vi "hoofdprogramma.vi"   [LabVIEW 2019]
uses:
  <vilib>/myRIO/Common/Instrument Driver Framework/Utilities/typedefs/Analog Scaling Constants.ctl
  <vilib>/myRIO/Common/Instrument Driver Framework/Utilities/typedefs/Analog Scaling Constants List.ctl
  <vilib>/myRIO/Common/Instrument Driver Framework/myRIO v1.0/AO/typedefs/AO Channels Enum.ctl
  <vilib>/myRIO/Common/Instrument Driver Framework/myRIO v1.0/AO/typedefs/AO Channels List.ctl
  <vilib>/myRIO/Common/Instrument Driver Framework/Utilities/typedefs/Generic FPGA Reference.ctl
  <vilib>/myRIO/Common/Instrument Driver Framework/Utilities/typedefs/myRIO v1.0 Reference.ctl
  <vilib>/myRIO/Common/Instrument Driver Framework/Utilities/typedefs/Hardware Version Enum.ctl
  <vilib>/myRIO/Common/Instrument Driver Framework/Utilities/typedefs/myRIO Generic Hardware Reference.ctl
  <vilib>/myRIO/Instrument Drivers/Onboard IO/AO/typedefs/AO Reference.ctl
  <vilib>/myRIO/Instrument Drivers/Onboard IO/AO/AO.lvlib
  <vilib>/myRIO/Instrument Drivers/Onboard IO/AO/vis/Write.vi
  <vilib>/userDefined/High Color/nirio_resource_hc.ctl
  <vilib>/myRIO/Common/Instrument Driver Framework/myRIO v1.0/AO/vis/myRIO v1.1 Open AO.vi
  <vilib>/myRIO/Instrument Drivers/Onboard IO/AO/vis/myRIO AO Open.xnode
  <vilib>/myRIO/Common/Instrument Driver Framework/Utilities/vis/Is FPGA Ref Available.vi
  <vilib>/myRIO/Express VI/Onboard IO/AO/AO Express VI.xnode
  <vilib>/myRIO/Common/Instrument Driver Framework/myRIO v1.0/DIO/typedefs/DIO Channels Enum.ctl
  <vilib>/myRIO/Common/Instrument Driver Framework/myRIO v1.0/DIO/typedefs/DIO Channels List.ctl
  <vilib>/myRIO/Instrument Drivers/Onboard IO/DIO/typedefs/DIO Reference.ctl
  <vilib>/myRIO/Instrument Drivers/Onboard IO/DIO/DIO.lvlib
  <vilib>/myRIO/Instrument Drivers/Onboard IO/DIO/vis/myRIO DIO Open.xnode
  <vilib>/myRIO/Common/Instrument Driver Framework/myRIO v1.0/DIO/vis/myRIO v1.1 Open DIO.vi
  <vilib>/myRIO/Instrument Drivers/Onboard IO/DIO/vis/Write.vi
  <vilib>/myRIO/Express VI/Onboard IO/DO/DO Express VI.xnode
  <vilib>/myRIO/Express VI/Onboard IO/DI/DI Express VI.xnode
  <vilib>/myRIO/Instrument Drivers/Onboard IO/DIO/vis/Read.vi
  interface.vi
types:
  T1 = typedef "DIO.lvlib/DIO Reference.ctl" = cluster{"myRIO Reference":T2, "DIO Channels List":T6}
  T2 = typedef "myRIO Generic Hardware Reference.ctl" = cluster{"myRIO Model":T3, "myRIO Hardware Reference":T4}
  T3 = typedef "Hardware Version Enum.ctl" = enum16{"Unknown", "myRIO-1900", "myRIO-1950", "roboRIO", "NI ELVIS RIO CM", "ELVIS III"}
  T4 = typedef "myRIO v1.0 Reference.ctl" = cluster{"Generic FPGA Reference":T5, "Allow multiple opens":bool}
  T5 = typedef "Generic FPGA Reference.ctl" = refnum<k20>
  T6 = typedef "DIO Channels List.ctl" = T7[]
  T7 = typedef "DIO Channels Enum.ctl" = enum16{"Not Connected", "C/DIO0", "C/DIO1", "C/DIO2", "C/DIO3", "C/DIO4", "C/DIO5", "C/DIO6", "C/DIO7", "A/DIO0", "A/DIO1", "A/DIO2", "A/DIO3", "A/DIO4", "A/DIO5", "A/DIO6", "A/DIO7", "A/DIO8", "A/DIO9", "A/DIO10", "A/DIO11", "A/DIO12", "A/DIO13", "A/DIO14", "A/DIO15", "A/DIO16", "A/DIO17", "A/DIO18", "A/DIO19", "B/DIO0", "B/DIO1", "B/DIO2", "B/DIO3", "B/DIO4", "B/DIO5", "B/DIO6", "B/DIO7", "B/DIO8", "B/DIO9", "B/DIO10", "B/DIO11", "B/DIO12", "B/DIO13", "B/DIO14", "B/DIO15", "B/DIO16", "B/DIO17", "B/DIO18", "B/DIO19", "LED0", "LED1", "LED2", "LED3", "Button0", "DIO/DIO0", "DIO/DIO1", "DIO/DIO2", "DIO/DIO3", "DIO/DIO4", "DIO/DIO5", "DIO/DIO6", "DIO/DIO7", "DIO/DIO8", "DIO/DIO9", "SPI/CS0", "SPI/CS1", "SPI/CS2", "SPI/CS3", "LED RADIO (Green)", "LED RADIO (Red)", "LED COMM (Green)", "LED COMM (Red)", "LED MODE (Green)", "LED MODE (Red)"}
  T8 = typedef "nirio_resource_hc.ctl" = tag
  T9 = typedef "AO.lvlib/AO Reference.ctl" = cluster{"myRIO Reference":T2, "AO Channel List":T10, "AO Scaling Constant List":T12}
  T10 = typedef "AO Channels List.ctl" = T11[]
  T11 = typedef "AO Channels Enum.ctl" = enum16{"Not Connected", "AudioOut/Left", "AudioOut/Right", "C/AO0", "C/AO1", "A/AO0", "A/AO1", "B/AO0", "B/AO1"}
  T12 = typedef "Analog Scaling Constants List.ctl" = T13[]
  T13 = typedef "Analog Scaling Constants.ctl" = cluster{"LSB Weight (Volts)":dbl, "Offset (Volts)":dbl, "Signed?":bool}
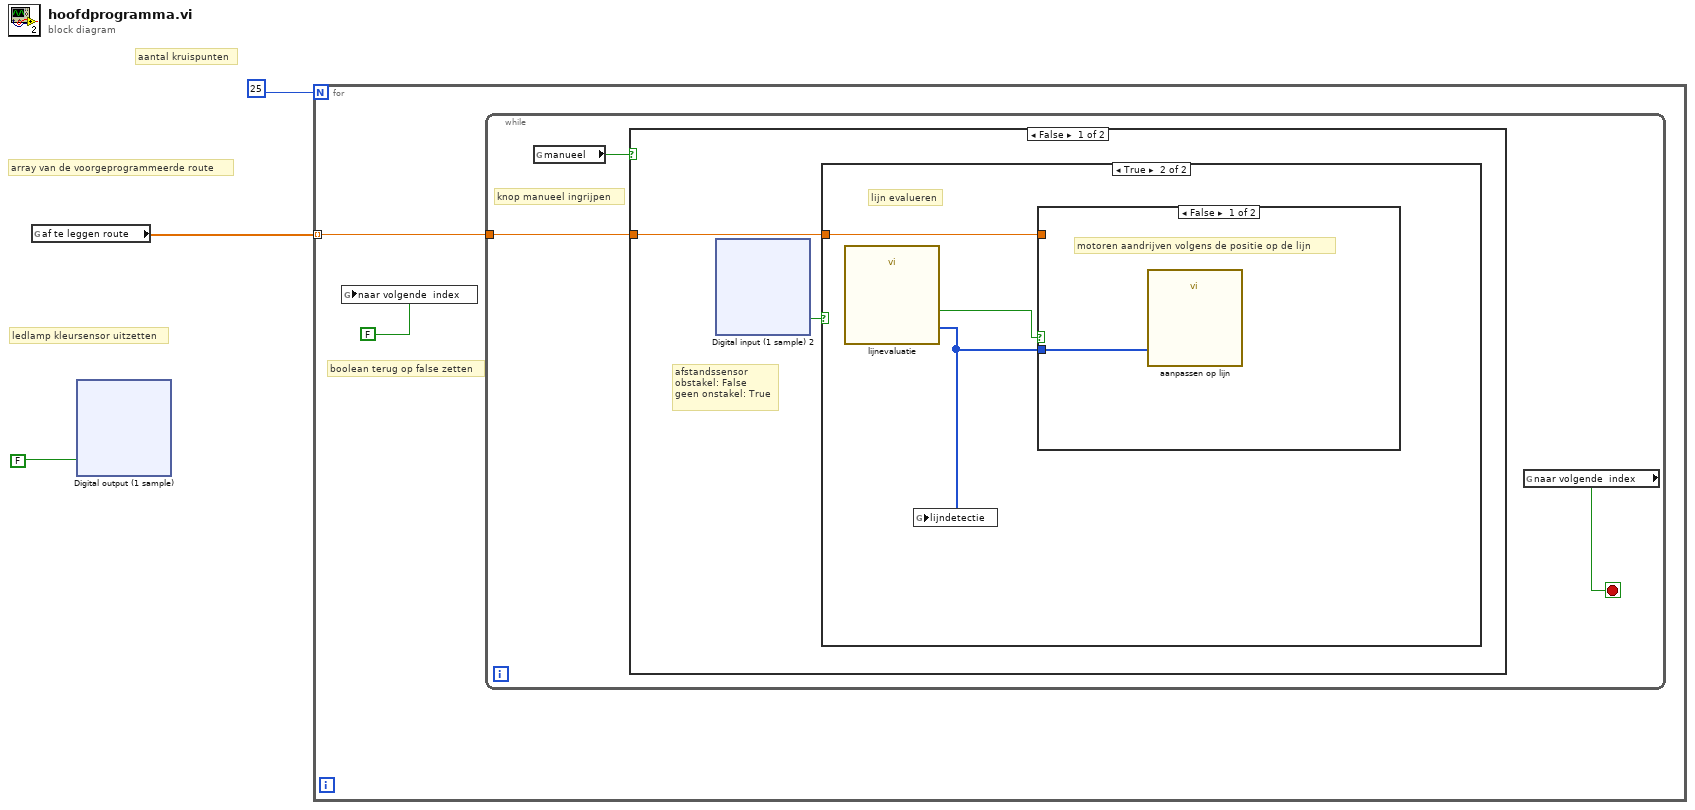
[diagram p0: block diagram]
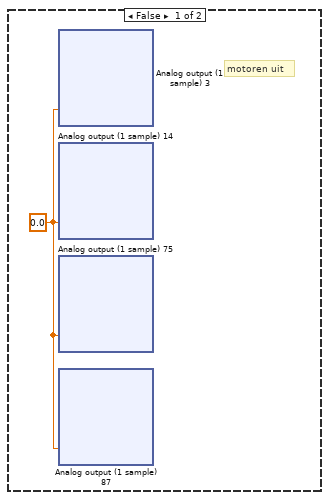
[diagram p2: hidden frame]
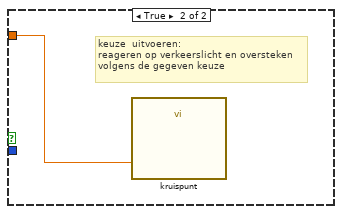
[diagram p3: hidden frame]
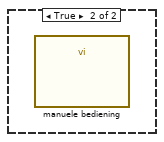
[diagram p4: hidden frame]
diagram:
  # "array van de voorgeprogrammeerde route"
  # "aantal kruispunten"
  # "ledlamp kleursensor uitzetten"
  n1 = global read "interface.vi" "af te leggen route"() -> (w1:dbl[])
  n2 = xnode "Digital output (1 sample)"("A/DIO2 (Pin 15)"=FALSE) -> ()  [unwired: 1 in, 1 out]
  n3 = for {
    N: 25 -> [_]
    tunnel: w1 -> [w5] mode=indexing
    # "boolean terug op false zetten"
    n4 = global write "interface.vi" "naar volgende  index"(FALSE) -> ()
    n5 = while {
      tunnel: w5 -> [w8]
      stop <- w6 stop-if-true
      # "knop manueel ingrijpen"
      n6 = global read "interface.vi" "manueel"() -> (w7:bool)
      n7 = case shown="False" w7 {
        tunnel: w8 -> [w9 _]
        frame False {
          # "afstandssensor\nobstakel: False\ngeen onstakel: True"
          n8 = xnode "Digital input (1 sample) 2"() -> ("A/DIO1 (Pin 13)"=w10:bool)  [unwired: 1 in, 1 out]
          n9 = case shown="True" w10 {
            tunnel: w9 -> [_ w197]
            frame False {
              w46 = 0.0
              # "motoren uit"
              n10 = xnode "Analog output (1 sample) 3"("A/AO0 (Pin 2)"=w46) -> ()  [unwired: 1 in, 1 out]
              n11 = xnode "Analog output (1 sample) 14"("A/AO1 (Pin 4)"=w46) -> ()  [unwired: 1 in, 1 out]
              n12 = xnode "Analog output (1 sample) 75"("B/AO0 (Pin 2)"=w46) -> ()  [unwired: 1 in, 1 out]
              n13 = xnode "Analog output (1 sample) 87"("B/AO1 (Pin 4)"=w46) -> ()  [unwired: 1 in, 1 out]
            }
            frame True {
              # "lijn evalueren"
              n14 = call "lijnevaluatie.vi"() -> ("digitaal lijn 0-1"=w195:i32[], "stopstreep indicator"=w196:bool)  [unwired: 8 in, 2 out]
              n15 = global write "interface.vi" "lijndetectie"(w195) -> ()
              n16 = case shown="False" w196 {
                tunnel: w197 -> [_ w199]
                tunnel: w195 -> [w198 _]
                frame False {
                  # "motoren aandrijven volgens de positie op de lijn"
                  n17 = call "aanpassen op lijn.vi"("digitaal lijn"=w198) -> ()  [unwired: 10 in, 1 out]
                }
                frame True {
                  # "keuze  uitvoeren:\nreageren op verkeerslicht en oversteken\nvolgens de gegeven keuze"
                  n18 = call "kruispunt.vi"("keuze 1,2 of 3"=w199) -> ()  [unwired: 11 in]
                }
              }
            }
          }
        }
        frame True {
          n19 = call "manuele bediening.vi"() -> ()  [unwired: 12 in]
        }
      }
      n20 = global read "interface.vi" "naar volgende  index"() -> (w6:bool)
    }
  }
